vi "SF2 Rational Interpolation.vi"(11 "Time":u32) -> (3 "Quat (out)":T1)   [LabVIEW 2016]
uses:
  <vilib>/Analysis/NI_AALPro.lvlib
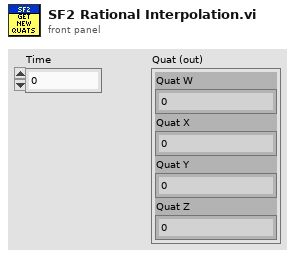
[diagram p1: front panel]
types:
  T1 = cluster{"Quat W":dbl, "Quat X":dbl, "Quat Y":dbl, "Quat Z":dbl}
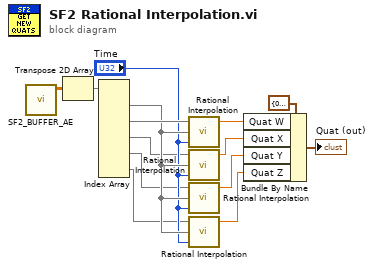
[diagram p0: block diagram]
diagram:
  n1 = call "SF2_BUFFER_AE.vi"() -> ("SF2 Buffer (out)"=w2:dbl[][])  [unwired: 11 in]
  n2 = Transpose 2D Array(2D array=w2) -> (transposed array=w1:dbl[][])
  n3 = Index Array(array=w1) -> (element #1=w13:dbl[], element #2=w14:dbl[], element #3=w11:dbl[], element #4=w10:dbl[], element #5=w9:dbl[])  [unwired: 10 in]
  n4 = call <vilib>:"Rational Interpolation.vi"("x value"="Time", "X"=w13, "Y"=w14) -> ("interpolation value"=w7:dbl)  [unwired: 2 out]
  n5 = call <vilib>:"Rational Interpolation.vi"("x value"="Time", "X"=w13, "Y"=w11) -> ("interpolation value"=w6:dbl)  [unwired: 2 out]
  n6 = call <vilib>:"Rational Interpolation.vi"("x value"="Time", "X"=w13, "Y"=w10) -> ("interpolation value"=w5:dbl)  [unwired: 2 out]
  n7 = call <vilib>:"Rational Interpolation.vi"("x value"="Time", "X"=w13, "Y"=w9) -> ("interpolation value"=w4:dbl)  [unwired: 2 out]
  n8 = Bundle By Name(cluster=T1 {"Quat W"=0.0, "Quat X"=0.0, "Quat Y"=0.0, "Quat Z"=0.0} ("qa"), "Quat W"=w7, "Quat X"=w6, "Quat Y"=w5, "Quat Z"=w4) -> (→"Quat (out)":T1)
